vi "tm3samp_01a_snapbutton.vi"() -> ()   [LabVIEW 2011]
panel:
  in  "Quit":bool
  in  "About":bool
  in  "Snap":bool
  out "Image":u16[][](graph)
  out "Error Out":errorcluster
  # "This is a method to capture multiple frames without reallocating the buffer."
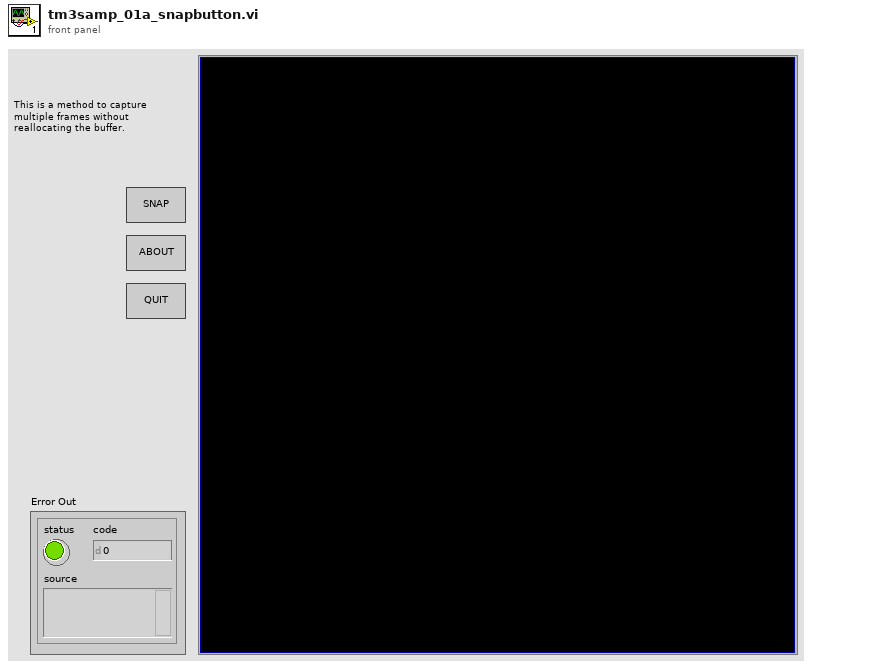
[diagram p1: front panel]
types:
  T1 = cluster{"height":u32, "width":u32, "datatype":u32}
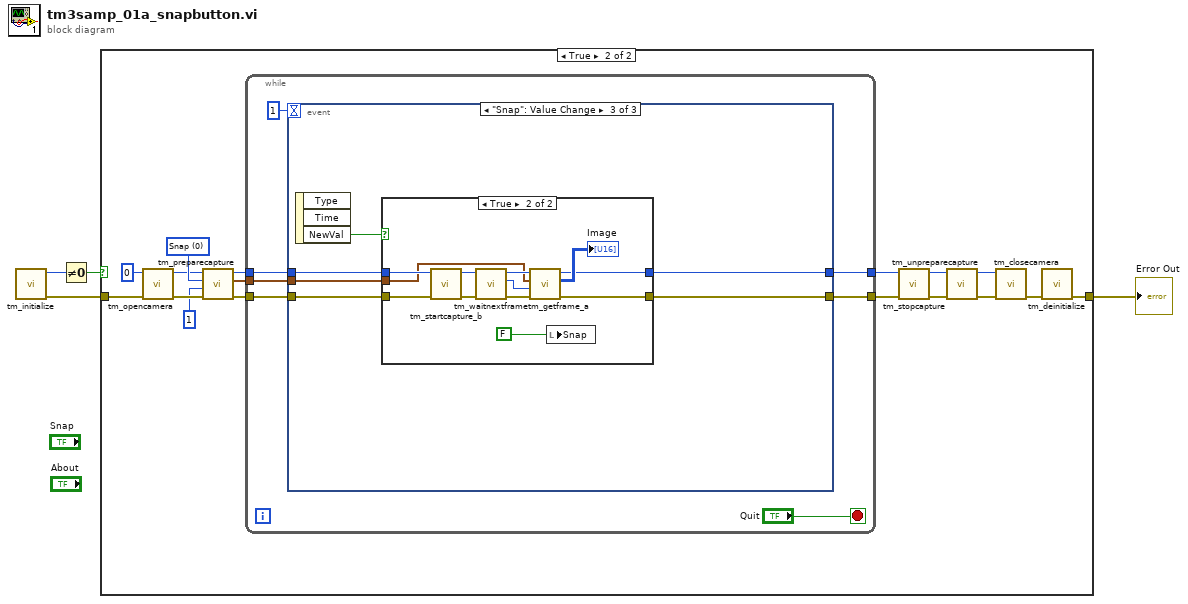
[diagram p0: block diagram]
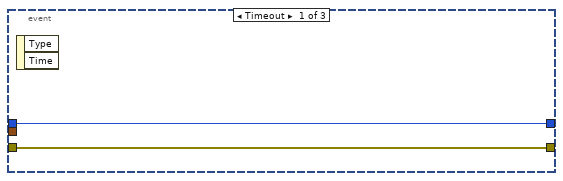
[diagram p3: hidden frame]
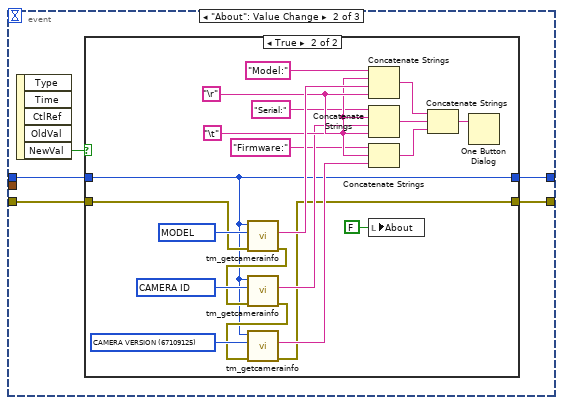
[diagram p4: hidden frame]
diagram:
  n1 = call <userlib>:"tm_initialize.vi"() -> ("error out"=w1:errorcluster, "Number Of Cameras"=w2:u32)  [unwired: 8 in, 2 out]
  n2 = Not Equal To 0?(x=w2) -> (x != 0?=w4:bool)
  n3 = case shown="True" w4 {
    tunnel: w1 -> [w5 w22]
    tunnel: [w5 w19] -> w3
    frame False {
    }
    frame True {
      w14 = 0 items=["Snap", "Sequence"] ("Capture mode")
      n4 = call <userlib>:"tm_opencamera.vi"("error in (no error)"=w22, "Camera Index"=u32 0) -> ("error out"=w12:errorcluster, "Handle out"=w13:u32)  [unwired: 7 in, 1 out]
      n5 = call <userlib>:"tm_preparecapture.vi"("error in (no error)"=w12, "Frames"=1, "Capture mode"=w14, "Handle in"=w13) -> ("error out"=w8:errorcluster, "Buffer Info"=w9:T1, "Handle out"=w10:u32)  [unwired: 4 in, 1 out]
      n6 = while {
        tunnel: w10 -> [w27]
        tunnel: w9 -> [w28]
        tunnel: w8 -> [w29]
        tunnel: [w26] -> w7
        tunnel: [w25] -> w6
        stop <- "Quit" stop-if-true
        n7 = event shown="[2] \"Snap\": Value Change" {
          selector: _ -> [_ _ _]
          dyn-events: _ -> [_ _ _]
          timeout: 1 -> [_ _ _]
          tunnel: w29 -> [w30 w35 w65]
          tunnel: w27 -> [w31 w34 w63]
          tunnel: w28 -> [_ _ w62]
          tunnel: [w31 w32 w61] -> w26
          tunnel: [w30 w33 w60] -> w25
          event Timeout {
            n8 = event-data() -> ()  [unwired: 1 in, 2 out]
          }
          event "About": Value Change {
            n9 = event-data() -> ("NewVal"=w36:bool)  [unwired: 1 in, 4 out]
            n10 = case shown="True" w36 {
              tunnel: w35 -> [w37 w42]
              tunnel: w34 -> [w38 w40]
              tunnel: [w37 w41] -> w33
              tunnel: [w38 w40] -> w32
              frame False {
              }
              frame True {
                w51 = "\t"
                w52 = "\r"
                w59 = u32 67109122 items=["BUS"=67109121, "CAMERA ID"=67109122, "VENDOR"=67109123, "MODEL"=67109124, "CAMERA VERSION"=67109125, "DRIVER VERSION"=67109126, "MODULE VERSIOIN"=67109127, "DCAMAPI VERSION"=67109128] ("Info ID")
                w58 = u32 67109125 items=["BUS"=67109121, "CAMERA"=67109122, "VENDOR"=67109123, "MODEL"=67109124, "CAMERA VERSION"=67109125, "DRIVER VERSION"=67109126, "MODULE VERSIOIN"=67109127, "DCAMAPI VERSION"=67109128] ("Info ID")
                w55 = u32 67109124 items=["BUS"=67109121, "CAMERA"=67109122, "VENDOR"=67109123, "MODEL"=67109124, "CAMERA VERSION"=67109125, "DRIVER VERSION"=67109126, "MODULE VERSIOIN"=67109127, "DCAMAPI VERSION"=67109128] ("Info ID")
                n11 = call <userlib>:"tm_getcamerainfo.vi"("error in (no error)"=w42, "Info ID"=w55, "Handle in"=w40) -> ("error out"=w56:errorcluster, "String"=w53:string)  [unwired: 6 in, 1 out]
                n12 = call <userlib>:"tm_getcamerainfo.vi"("error in (no error)"=w56, "Info ID"=w59, "Handle in"=w40) -> ("error out"=w57:errorcluster, "String"=w49:string)  [unwired: 6 in, 1 out]
                n13 = call <userlib>:"tm_getcamerainfo.vi"("error in (no error)"=w57, "Info ID"=w58, "Handle in"=w40) -> ("error out"=w41:errorcluster, "String"=w50:string)  [unwired: 6 in, 1 out]
                n14 = Concatenate Strings("Model:", w51, w53, w52) -> (w46:string)
                n15 = Concatenate Strings("Serial:", w51, w49, w52) -> (w45:string)
                n16 = Concatenate Strings("Firmware:", w51, w50) -> (w44:string)
                n17 = local write "About"(FALSE ("About")) -> ()
                n18 = Concatenate Strings(w46, w45, w44) -> (w43:string)
                n19 = One Button Dialog(message=w43) -> ()  [unwired: 1 in, 1 out]
              }
            }
          }
          event "Snap": Value Change {
            n20 = event-data() -> ("NewVal"=w64:bool)  [unwired: 1 in, 2 out]
            n21 = case shown="True" w64 {
              tunnel: w65 -> [w66 w72]
              tunnel: w63 -> [w67 w73]
              tunnel: w62 -> [_ w71]
              tunnel: [w67 w70] -> w61
              tunnel: [w66 w69] -> w60
              frame False {
              }
              frame True {
                n22 = call <userlib>:"tm_startcapture_b.vi"("error in (no error)"=w72, "Handle in"=w73) -> ("error out"=w78:errorcluster, "Handle out"=w77:u32)  [unwired: 8 in]
                n23 = call <userlib>:"tm_waitnextframe.vi"("error in (no error)"=w78, "Handle in"=w77) -> ("error out"=w76:errorcluster, "Frame Index"=w74:i32, "Handle out"=w75:u32)  [unwired: 6 in, 1 out]
                n24 = call <userlib>:"tm_getframe_a.vi"("error in (no error)"=w76, "Frame Index"=w74, "Buffer Info"=w71, "Handle in"=w75) -> ("error out"=w69:errorcluster, "Data 16"=→"Image":u16[][], "Handle out"=w70:u32)  [unwired: 3 in, 2 out]
                n25 = local write "Snap"(FALSE) -> ()
              }
            }
          }
        }
      }
      n26 = call <userlib>:"tm_stopcapture.vi"("error in (no error)"=w6, "Handle in"=w7) -> ("error out"=w15:errorcluster, "Handle out"=w16:u32)  [unwired: 8 in]
      n27 = call <userlib>:"tm_unpreparecapture.vi"("error in (no error)"=w15, "Handle in"=w16) -> ("error out"=w18:errorcluster, "Handle out"=w17:u32)  [unwired: 8 in]
      n28 = call <userlib>:"tm_closecamera.vi"("error in (no error)"=w18, "Handle in"=w17) -> ("error out"=w20:errorcluster)  [unwired: 9 in]
      n29 = call <userlib>:"tm_deinitialize.vi"("error in (no error)"=w20) -> ("error out"=w19:errorcluster)  [unwired: 10 in]
    }
  }
  "Error Out" <- w3
